vi "PRESSURE_TRANSMITTER.vi"(2 "Low Value Set-point":dbl, 3 "Input":dbl, 4 "High Value Set-point":dbl) -> (0 "Low Limit":bool, 1 "High Limit":bool)   [LabVIEW 2014]
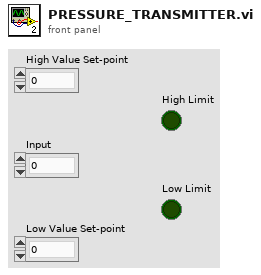
[diagram p1: front panel]
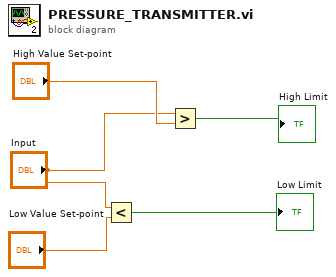
[diagram p0: block diagram]
diagram:
  n1 = Less?(x="Input", y="Low Value Set-point") -> (x < y?=→"Low Limit":bool)
  n2 = Greater?(x="Input", y="High Value Set-point") -> (0:→"High Limit":bool)
